vi "ZeroMQ_ACS3.vi"() -> ()   [LabVIEW 2018]
uses:
  <vilib>/addons/zeromq/socket_type.ctl
  <vilib>/addons/zeromq/socket_options.ctl
  <vilib>/addons/zeromq/zeromq.lvlib
  <vilib>/addons/zeromq/zmq_socket.lvclass
  <vilib>/addons/zeromq/zmq_context.lvclass
panel:
  out "error out 4":errorcluster
  in  "stop 4":bool
  out "command 2":string
  out "reply":string
  out "error out 2":errorcluster
  out "ADDRESS SUB":string
  out "response sub":string
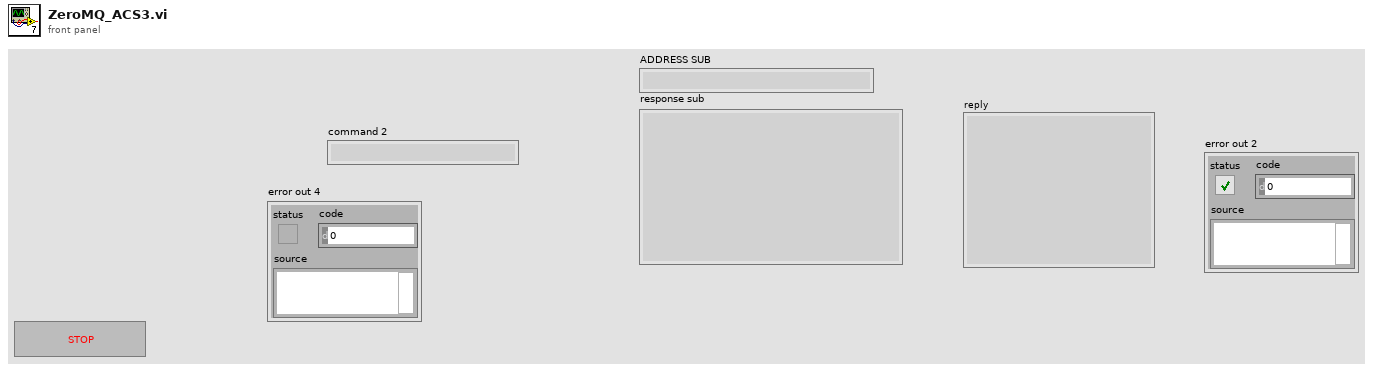
[diagram p1: front panel]
types:
  T1 = typedef "zeromq.lvlib/socket_options.ctl" = enum8{"NONE", "ZMQ_HWM", "<2>", "ZMQ_SWAP", "ZMQ_AFFINITY", "ZMQ_ROUTING_ID", "ZMQ_SUBSCRIBE", "ZMQ_UNSUBSCRIBE", "ZMQ_RATE", "ZMQ_RECOVERY_IVL", "ZMQ_MCAST_LOOP", "ZMQ_SNDBUF", "ZMQ_RCVBUF", "ZMQ_RCVMORE", "ZMQ_FD", "ZMQ_EVENTS", "ZMQ_TYPE", "ZMQ_LINGER", "ZMQ_RECONNECT_IVL", "ZMQ_BACKLOG", "ZMQ_RECOVERY_IVL_MSEC", "ZMQ_RECONNECT_IVL_MAX", "ZMQ_MAXMSGSIZE", "ZMQ_SNDHWM", "ZMQ_RCVHWM", "ZMQ_MULTICAST_HOPS", "<26>", "ZMQ_RCVTIMEO", "ZMQ_SNDTIMEO", "<29>", "<30>", "ZMQ_IPV4ONLY", "ZMQ_LAST_ENDPOINT", "ZMQ_ROUTER_MANDATORY", "ZMQ_TCP_KEEPALIVE", "ZMQ_TCP_KEEPALIVE_CNT", "ZMQ_TCP_KEEPALIVE_IDLE", "ZMQ_TCP_KEEPALIVE_INTVL", "ZMQ_TCP_ACCEPT_FILTER", "ZMQ_IMMEDIATE", "ZMQ_XPUB_VERBOSE", "ZMQ_ROUTER_RAW", "ZMQ_IPV6", "ZMQ_MECHANISM", "ZMQ_PLAIN_SERVER", "ZMQ_PLAIN_USERNAME", "ZMQ_PLAIN_PASSWORD", "ZMQ_CURVE_SERVER", "ZMQ_CURVE_PUBLICKEY", "ZMQ_CURVE_SECRETKEY", "ZMQ_CURVE_SERVERKEY", "ZMQ_PROBE_ROUTER", "ZMQ_REQ_CORRELATE", "ZMQ_REQ_RELAXED", "ZMQ_CONFLATE", "ZMQ_ZAP_DOMAIN", "ZMQ_ROUTER_HANDOVER", "ZMQ_TOS", "ZMQ_IPC_FILTER_PID", "ZMQ_IPC_FILTER_UID", "ZMQ_IPC_FILTER_GID", "ZMQ_CONNECT_ROUTING_ID", "ZMQ_GSSAPI_SERVER", "ZMQ_GSSAPI_PRINCIPAL", "ZMQ_GSSAPI_SERVICE_PRINCIPAL", "ZMQ_GSSAPI_PLAINTEXT", "ZMQ_HANDSHAKE_IVL", "<67>", "ZMQ_SOCKS_PROXY", "ZMQ_XPUB_NODROP", "ZMQ_BLOCKY", "ZMQ_XPUB_MANUAL", "ZMQ_XPUB_WELCOME_MSG", "ZMQ_STREAM_NOTIFY", "ZMQ_INVERT_MATCHING", "ZMQ_HEARTBEAT_IVL", "ZMQ_HEARTBEAT_TTL", "ZMQ_HEARTBEAT_TIMEOUT", "ZMQ_XPUB_VERBOSER", "ZMQ_CONNECT_TIMEOUT", "ZMQ_TCP_MAXRT", "ZMQ_THREAD_SAFE", "<82>", "<83>", "ZMQ_MULTICAST_MAXTPDU", "ZMQ_VMCI_BUFFER_SIZE", "ZMQ_VMCI_BUFFER_MIN_SIZE", "ZMQ_VMCI_BUFFER_MAX_SIZE", "ZMQ_VMCI_CONNECT_TIMEOUT", "ZMQ_USE_FD", "ZMQ_GSSAPI_PRINCIPAL_NAMETYPE", "ZMQ_GSSAPI_SERVICE_PRINCIPAL_NAMETYPE", "ZMQ_BINDTODEVICE", "ZMQ_ZAP_ENFORCE_DOMAIN", "ZMQ_LOOPBACK_FASTPATH", "ZMQ_METADATA", "ZMQ_MULTICAST_LOOP", "ZMQ_ROUTER_NOTIFY"}
  T2 = typedef "zeromq.lvlib/socket_type.ctl" = enum8{"ZMQ_PAIR", "ZMQ_PUB", "ZMQ_SUB", "ZMQ_REQ", "ZMQ_REP", "ZMQ_DEALER", "ZMQ_ROUTER", "ZMQ_PULL", "ZMQ_PUSH", "ZMQ_XPUB", "ZMQ_XSUB", "ZMQ_STREAM", "ZMQ_SERVER", "ZMQ_CLIENT", "ZMQ_RADIO", "ZMQ_DISH", "ZMQ_GATHER", "ZMQ_SCATTER", "ZMQ_DGRAM"}
  T3 = cluster{"ID":u32, "Address":string, "Service Name 1":string, "Service Name 2":string, "queue TX":refnum<queue>, "queue RX":refnum<queue>, "Port 1":u32, "Port 2":u32}
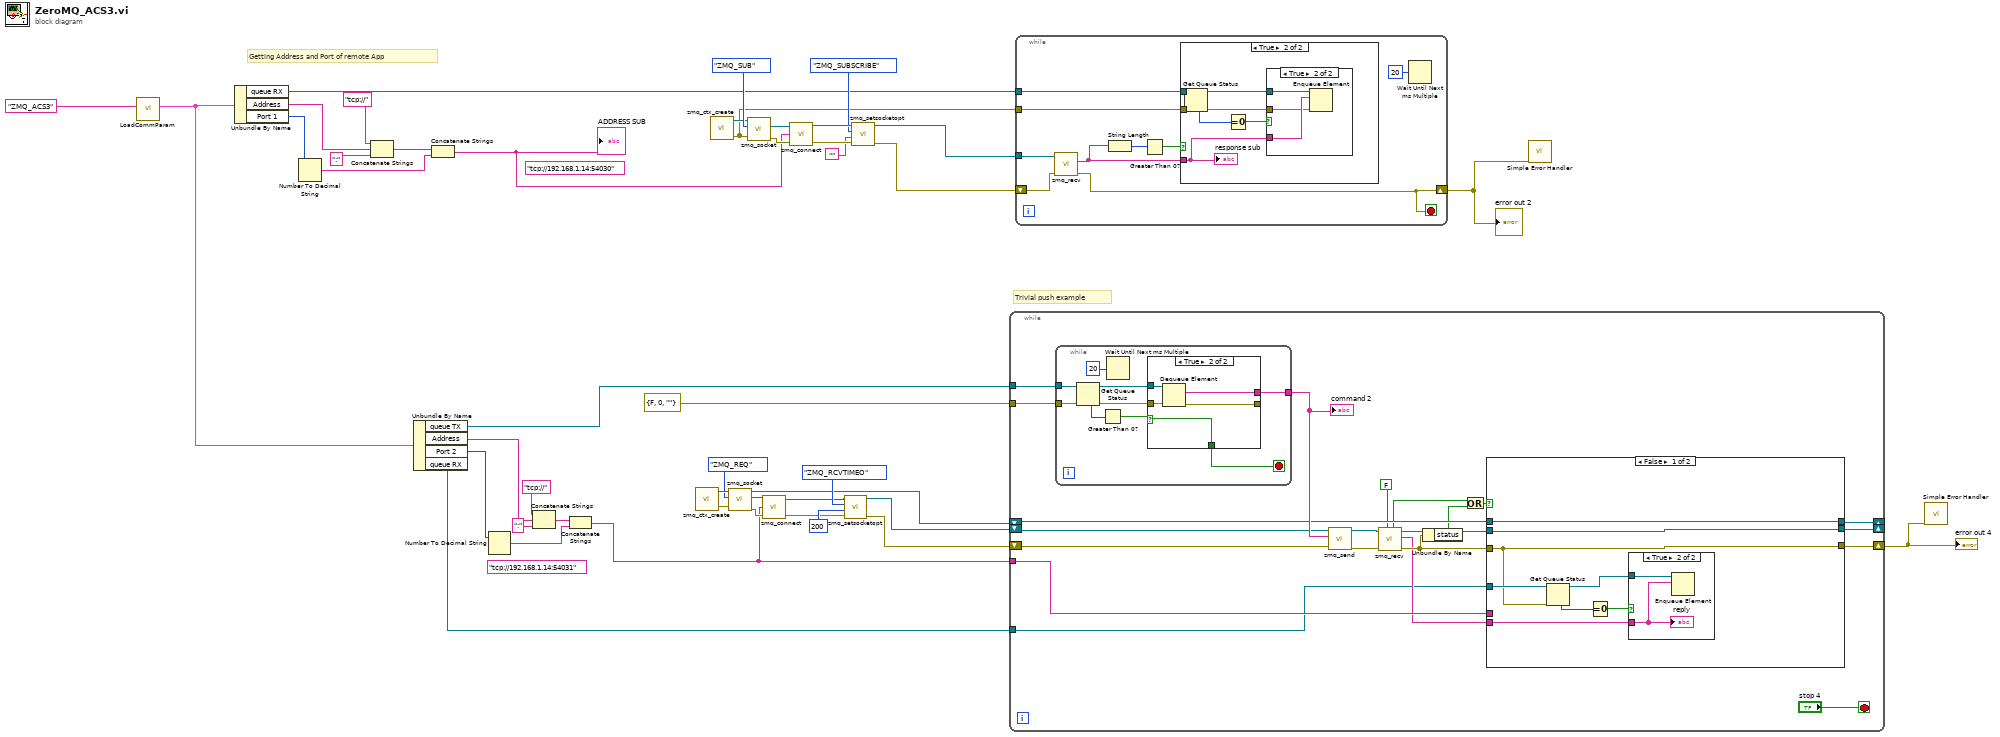
[diagram p0: block diagram]
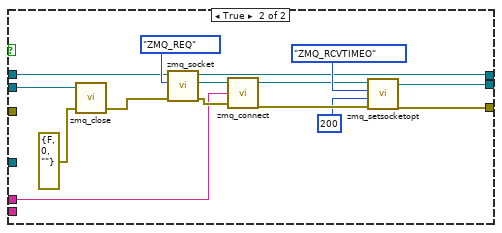
[diagram p3: hidden frame]
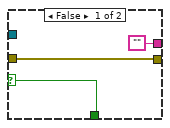
[diagram p4: hidden frame]
diagram:
  (unwired) "tcp://192.168.1.14:54031" ("endpoint")
  (unwired) "tcp://192.168.1.14:54030" ("endpoint")
  # "Trivial push example"
  # "Getting Address and Port of remote App"
  n1 = call "LoadCommParam.vi"("section name"="ZMQ_ACS3") -> ("output cluster"=w27:T3)  [unwired: 10 in]
  n2 = Unbundle By Name(w27) -> ("queue RX"=w33:refnum<queue>, "Address"=w25:string, "Port 1"=w32:u32)
  n3 = Number To Decimal String(number=w32) -> (decimal integer string=w31:string)  [unwired: 1 in]
  n4 = Concatenate Strings("tcp://" ("string"), w25, ":" ("string")) -> (w30:string)
  n5 = Unbundle By Name(w27) -> ("queue TX"=w16:refnum<queue>, "Address"=w18:string, "Port 2"=w17:u32, "queue RX"=w2:refnum<queue>)
  n6 = Concatenate Strings(w30, w31) -> (w35:string)
  "ADDRESS SUB" <- w35
  n7 = Number To Decimal String(number=w17) -> (decimal integer string=w22:string)  [unwired: 1 in]
  n8 = Concatenate Strings("tcp://" ("string"), w18, ":" ("string")) -> (w21:string)
  n9 = Concatenate Strings(w21, w22) -> (w10:string)
  n10 = call <vilib>:"zmq_ctx_create.vi"() -> ("error out"=w15:errorcluster, "context out"=w12:refnum<class "zmq_context.lvclass">)  [unwired: 4 in]
  n11 = call <vilib>:"zmq_ctx_create.vi"() -> ("error out"=w34:errorcluster, "context out"=w36:refnum<class "zmq_context.lvclass">)  [unwired: 4 in]
  n12 = call <vilib>:"zmq_socket.vi"("error in"=w15, "socket type"=socket_type."ZMQ_REQ", "context in"=w12) -> ("error out"=w13:errorcluster, "socket out"=w14:refnum<class "zmq_socket.lvclass">, "context out"=w5:refnum<class "zmq_context.lvclass">)  [unwired: 2 in]
  n13 = call <vilib>:"zmq_socket.vi"("error in"=w34, "socket type"=socket_type."ZMQ_SUB", "context in"=w36) -> ("error out"=w44:errorcluster, "socket out"=w37:refnum<class "zmq_socket.lvclass">)  [unwired: 2 in, 1 out]
  n14 = call <vilib>:"zmq_connect.vi"("error in"=w13, "endpoint"=w10, "socket in"=w14) -> ("error out"=w6:errorcluster, "socket out"=w7:refnum<class "zmq_socket.lvclass">)  [unwired: 1 in]
  n15 = call <vilib>:"zmq_connect.vi"("error in"=w44, "endpoint"=w35, "socket in"=w37) -> ("error out"=w42:errorcluster, "socket out"=w43:refnum<class "zmq_socket.lvclass">)  [unwired: 1 in]
  n16 = call <vilib>:"zmq_setsocketopt.vi"("error in"=w6, "value"=200 ("max queue size (-1, unlimited)"), "option"=socket_options."ZMQ_RCVTIMEO", "socket in"=w7) -> ("error out"=w3:errorcluster, "socket out"=w4:refnum<class "zmq_socket.lvclass">)  [unwired: 2 in]
  n17 = call <vilib>:"zmq_setsocketopt.vi"("error in"=w42, "value"="", "option"=socket_options."ZMQ_SUBSCRIBE", "socket in"=w43) -> ("error out"=w41:errorcluster, "socket out"=w40:refnum<class "zmq_socket.lvclass">)  [unwired: 2 in]
  n18 = while {
    tunnel: w16 -> [w66]
    tunnel: errorcluster {"status"=FALSE, "code"=0, "source"=""} ("error out") -> [w62]
    tunnel: w10 -> [w51]
    shift-right: [w50] -> _
    shift-left: w5 -> [w61]
    shift-right: [w49] -> _
    shift-left: w4 -> [w60]
    shift-right: [w63] -> w24
    shift-left: w3 -> [w48]
    tunnel: w2 -> [w46]
    stop <- "stop 4" stop-if-true
    n19 = while {
      tunnel: w66 -> [w99]
      tunnel: w62 -> [w98]
      tunnel: [w94] -> w65
      stop <- w93 stop-if-true
      n20 = Get Queue Status(queue=w99, error in (no error)=w98) -> (queue out=w95:refnum<queue>, error out=w96:errorcluster, # elements in queue=w100:i32)  [unwired: 1 in, 5 out]
      n21 = Greater Than 0?(x=w100) -> (x > 0?=w97:bool)
      n22 = Wait Until Next ms Multiple(millisecond multiple=u32 20) -> ()  [unwired: 1 out]
      n23 = case shown="True" w97 {
        selector: w97 -> [w101 w104]
        tunnel: w96 -> [w103 w108]
        tunnel: w95 -> [_ w107]
        tunnel: [w103 w106] -> _
        tunnel: ["" w105] -> w94
        tunnel: [w101 w104] -> w93
        frame False {
        }
        frame True {
          n24 = Dequeue Element(queue=w107, error in (no error)=w108) -> (element=w105:string, error out=w106:errorcluster)  [unwired: 1 in, 2 out]
        }
      }
    }
    "command 2" <- w65
    n25 = call <vilib>:"zmq_send.vi"("error in"=w48, "data"=w65, "socket in"=w60) -> ("error out"=w58:errorcluster, "socket out"=w59:refnum<class "zmq_socket.lvclass">)  [unwired: 4 in]
    n26 = call <vilib>:"zmq_recv.vi"("no block? (F)"=FALSE, "error in"=w58, "socket in"=w59) -> ("error out"=w53:errorcluster, "data"=w47:string, "socket out"=w52:refnum<class "zmq_socket.lvclass">, "timeout?"=w54:bool)  [unwired: 2 in, 1 out]
    n27 = Unbundle By Name(w53) -> ("status"=w55:bool)
    n28 = Or(x=w54, y=w55) -> (x .or. y?=w56:bool)
    n29 = case shown="False" w56 {
      tunnel: [w67 w79] -> w63
      tunnel: w61 -> [w73 w81]
      tunnel: w53 -> [w67 _]
      tunnel: w52 -> [w74 w82]
      tunnel: w51 -> [_ w80]
      tunnel: [w74 w78] -> w49
      tunnel: [w73 w77] -> w50
      tunnel: w47 -> [w69 _]
      tunnel: w46 -> [w68 _]
      frame False {
        n30 = Get Queue Status(queue=w68, error in (no error)=w67) -> (queue out=w70:refnum<queue>, # elements in queue=w72:i32)  [unwired: 1 in, 6 out]
        n31 = Equal To 0?(x=w72) -> (x = 0?=w71:bool)
        n32 = case shown="True" w71 {
          tunnel: w70 -> [_ w76]
          tunnel: w69 -> [_ w75]
          frame False {
          }
          frame True {
            n33 = Enqueue Element(queue=w76, element=w75) -> ()  [unwired: 2 in, 3 out]
            "reply" <- w75
          }
        }
      }
      frame True {
        n34 = call <vilib>:"zmq_close.vi"("error in"=errorcluster {"status"=FALSE, "code"=0, "source"=""}, "socket"=w82) -> ("error out"=w84:errorcluster)  [unwired: 3 in]
        n35 = call <vilib>:"zmq_socket.vi"("error in"=w84, "socket type"=socket_type."ZMQ_REQ", "context in"=w81) -> ("error out"=w90:errorcluster, "socket out"=w91:refnum<class "zmq_socket.lvclass">, "context out"=w77:refnum<class "zmq_context.lvclass">)  [unwired: 2 in]
        n36 = call <vilib>:"zmq_connect.vi"("error in"=w90, "endpoint"=w80, "socket in"=w91) -> ("error out"=w86:errorcluster, "socket out"=w87:refnum<class "zmq_socket.lvclass">)  [unwired: 1 in]
        n37 = call <vilib>:"zmq_setsocketopt.vi"("error in"=w86, "value"=200 ("max queue size (-1, unlimited)"), "option"=socket_options."ZMQ_RCVTIMEO", "socket in"=w87) -> ("error out"=w79:errorcluster, "socket out"=w78:refnum<class "zmq_socket.lvclass">)  [unwired: 2 in]
      }
    }
  }
  "error out 4" <- w24
  n38 = while {
    tunnel: w40 -> [w110]
    tunnel: w33 -> [w113]
    shift-right: [w116] -> w26
    shift-left: w41 -> [w117]
    tunnel: w34 -> [w111]
    stop <- w116 stop-if-true
    n39 = call <vilib>:"zmq_recv.vi"("error in"=w117, "socket in"=w110) -> ("error out"=w116:errorcluster, "data"=w112:string)  [unwired: 3 in, 3 out]
    n40 = String Length(string=w112) -> (length=w115:i32)
    n41 = Greater Than 0?(x=w115) -> (x > 0?=w114:bool)
    n42 = case shown="True" w114 {
      tunnel: w113 -> [_ w123]
      tunnel: w112 -> [_ w120]
      tunnel: w111 -> [_ w119]
      frame False {
      }
      frame True {
        n43 = Get Queue Status(queue=w123, error in (no error)=w119) -> (queue out=w121:refnum<queue>, error out=w118:errorcluster, # elements in queue=w124:i32)  [unwired: 1 in, 5 out]
        n44 = Equal To 0?(x=w124) -> (x = 0?=w122:bool)
        n45 = case shown="True" w122 {
          tunnel: w121 -> [_ w127]
          tunnel: w120 -> [_ w126]
          tunnel: w118 -> [_ w125]
          frame False {
          }
          frame True {
            n46 = Enqueue Element(queue=w127, element=w126, error in (no error)=w125) -> ()  [unwired: 1 in, 3 out]
          }
        }
        "response sub" <- w120
      }
    }
    n47 = Wait Until Next ms Multiple(millisecond multiple=u32 20) -> ()  [unwired: 1 out]
  }
  "error out 2" <- w26
  n48 = call <vilib>:"Simple Error Handler.vi"("error in (no error)"=w26) -> ()  [unwired: 4 in, 5 out]
  n49 = call <vilib>:"Simple Error Handler.vi"("error in (no error)"=w24) -> ()  [unwired: 4 in, 5 out]
